vi "MergeFiles.vi"(4 "Error In":errorcluster, 6 "MergeFileConfigIN":T1) -> (0 "sortie d'erreur":errorcluster)   [LabVIEW 2017]
uses:
  DefDeType/WhichPath.ctl
  DefDeType/MergeFileConfig.ctl
panel:
  out "AllWaveForms":waveform(dbl)[](graph)
  out "NortekWaveForms":waveform(dbl)[](graph)
  out "HexapodWaveForms":waveform(dbl)[](graph)
  out "QualisysWaveform":waveform(dbl)[](graph)
  out "ValiseWaveform":waveform(dbl)[](graph)
  out "Etat":string
  # "Merging files"
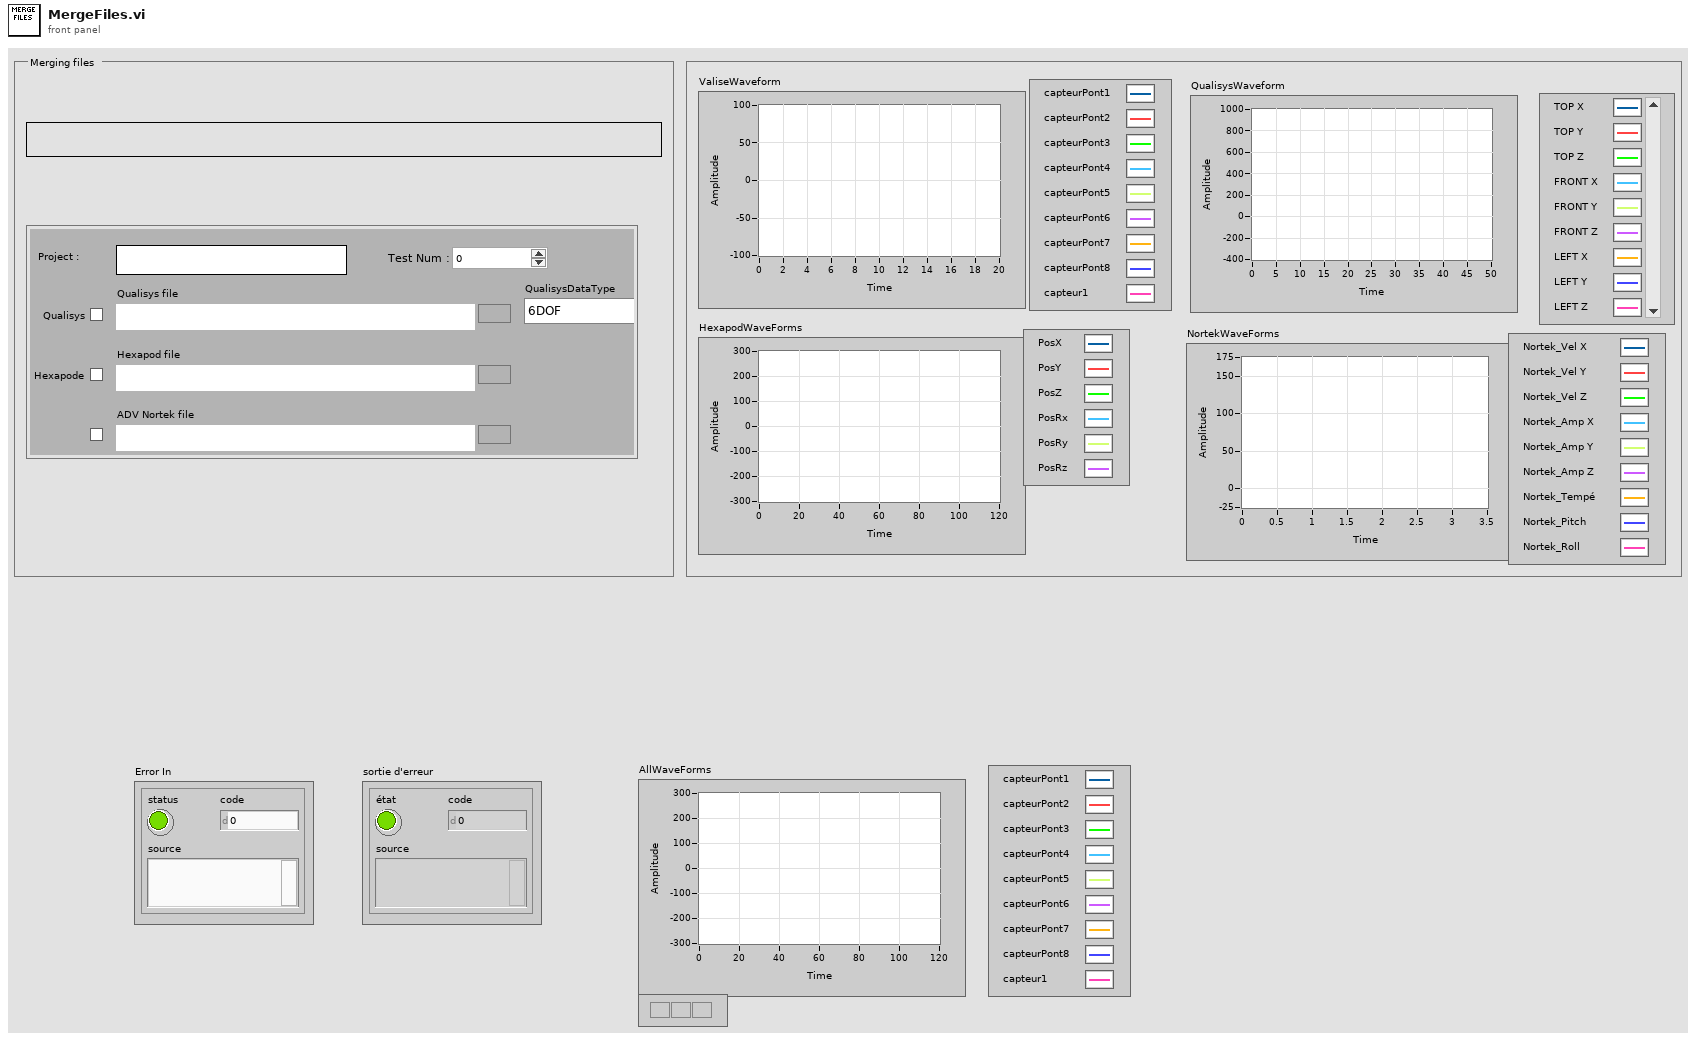
[diagram p1: front panel]
types:
  T1 = typedef "MergeFileConfig.ctl" = cluster{"Test Num : ":u32, "Project :":string, "Qualisys file":path, "Hexapod file":path, "ADV Nortek file":path, "QualisysDataType":enum16{"6DOF", "3DTracking", "6DOF + 3D"}, "Qualisys":bool, "Hexapode":bool, "ADV Nortek":bool}
  T2 = typedef "WhichPath.ctl" = enum16{"DossierProjet", "Config", "Meas", "MeasPCI", "MeasCRIO1", "MeasCRIO2", "MeasQualisys", "MeasHBM", "MeasTDMS", "Fig", "Res"}
  T3 = enum16{"open", "open or create", "create or replace", "create", "open (read-only)"}
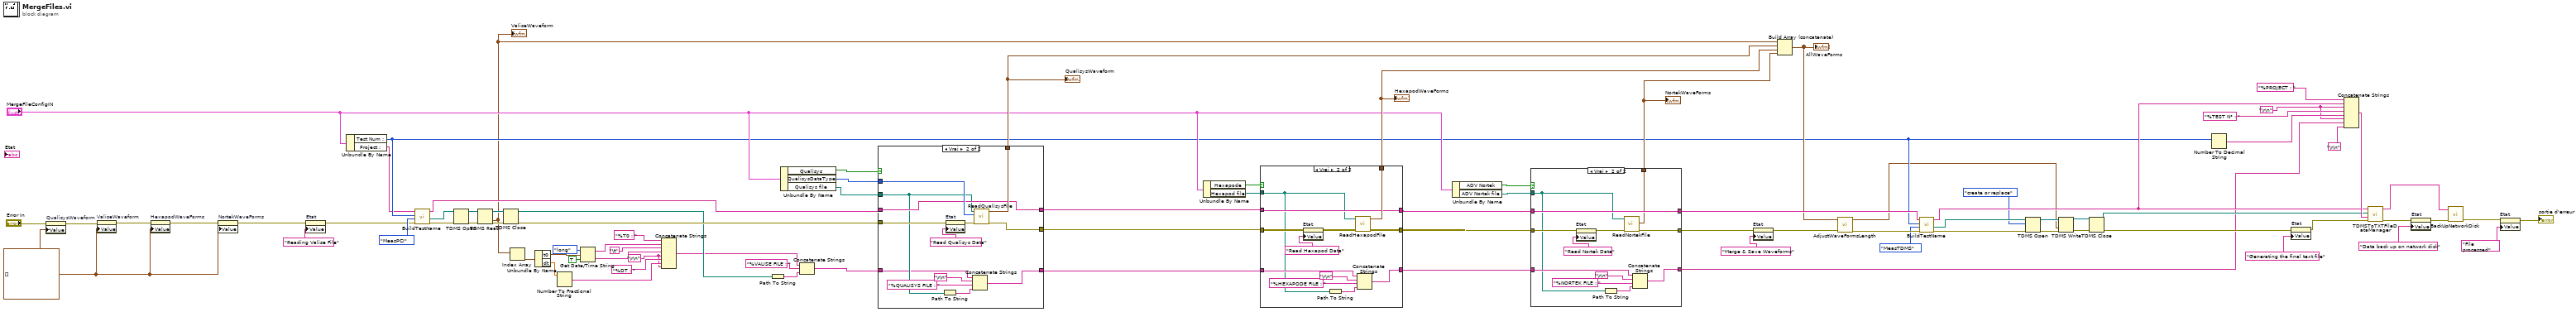
[diagram p0: block diagram]
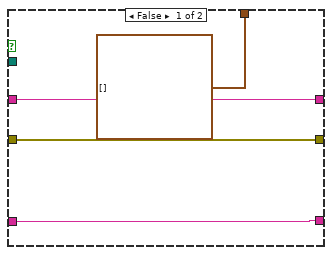
[diagram p2: hidden frame]
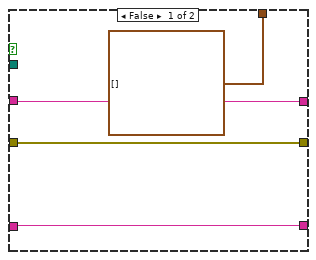
[diagram p3: hidden frame]
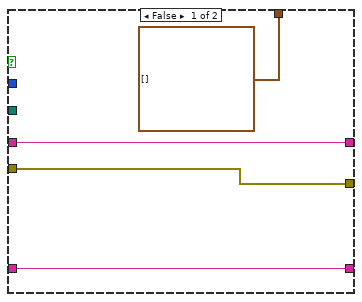
[diagram p4: hidden frame]
diagram:
  w3 = "\r\n"
  w77 = "\r\n"
  w58 = waveform(dbl)[] [] ("QualisysWaveforms")
  n1 = property on="QualisysWaveform" class="GraphWF (strict)"(error in="Error In", "Value"=w58) -> (error out=w82:errorcluster)  [unwired: 1 in, 1 out]
  n2 = property on="ValiseWaveform" class="GraphWF (strict)"(error in=w82, "Value"=w58) -> (error out=w66:errorcluster)  [unwired: 1 in, 1 out]
  n3 = property on="HexapodWaveForms" class="GraphWF (strict)"(error in=w66, "Value"=w58) -> (error out=w59:errorcluster)  [unwired: 1 in, 1 out]
  n4 = property on="NortekWaveForms" class="GraphWF (strict)"(error in=w59, "Value"=w58) -> (error out=w28:errorcluster)  [unwired: 1 in, 1 out]
  n5 = property on="Etat" class="Ch"(error in=w28, "Value"="Reading Valise File" ("Etat")) -> (error out=w29:errorcluster)  [unwired: 1 in, 1 out]
  n6 = Unbundle By Name("MergeFileConfigIN") -> ("Test Num :"=w33:u32, "Project :"=w23:string)
  n7 = call "BuildTestName.vi"("entrée d'erreur"=w29, "WhichPath?"=WhichPath."MeasPCI", "NextTestNum"=w33, "NomProjet"=w23) -> ("sortie d'erreur"=w30:errorcluster, "cheminProchainFichier"=w31:path, "NomProjetOut"=w34:string)  [unwired: 1 in, 1 out]
  n8 = TDMS Open(8:w30, 11:w31) -> (0:w38:errorcluster, 3:w37:refnum<k34>)  [unwired: 5 in]
  n9 = TDMS Read(0:w37, 11:w38) -> (4:w39:refnum<k34>, 10:w15:waveform(dbl)[], 15:w40:errorcluster)  [unwired: 6 in, 3 out]
  "ValiseWaveform" <- w15
  n10 = TDMS Close(8:w40, 11:w39) -> (0:w36:errorcluster, 3:w22:path)
  n11 = Index Array(array=w15) -> (element=w14:waveform(dbl))  [unwired: 1 in]
  n12 = Unbundle By Name(w14) -> ("t0"=w13:timestamp, "dt"=w6:dbl)
  n13 = Number To Fractional String(number=w6) -> (F-format string=w4:string)  [unwired: 3 in]
  n14 = Get Date/Time String(date format (0)=enum16{"short", "long", "abbreviated"}."long", seconds (now)=w13, want seconds? (F)=TRUE) -> (date string=w9:string, time string=w7:string)
  n15 = Concatenate Strings("%T0 : " ("Etat"), w9, "\t", w7, w3, "%DT : " ("Etat"), w4, w3) -> (w2:string)
  n16 = Path To String(path=w22) -> (string=w21:string)
  n17 = Unbundle By Name("MergeFileConfigIN") -> ("Qualisys"=w87:bool, "QualisysDataType"=w86:enum16{"6DOF", "3DTracking", "6DOF + 3D"}, "Qualisys file"=w27:path)
  n18 = Concatenate Strings(w2, "%VALISE FILE : " ("Etat"), w21) -> (w19:string)
  n19 = case shown="Vrai" w87 {
    tunnel: [w91 w105] -> w65
    tunnel: [w92 w99] -> w84
    tunnel: w34 -> [w92 w99]
    tunnel: w36 -> [w91 w100]
    tunnel: w86 -> [_ w104]
    tunnel: [waveform(dbl)[] [] ("QualisysWaveforms") w103] -> w62
    tunnel: w27 -> [_ w96]
    tunnel: w19 -> [w89 w94]
    tunnel: [w89 w93] -> w18
    frame False {
    }
    frame True {
      n20 = Path To String(path=w96) -> (string=w97:string)
      n21 = property on="Etat" class="Ch"(error in=w100, "Value"="Read Qualisys Data" ("Etat")) -> (error out=w101:errorcluster)  [unwired: 1 in, 1 out]
      n22 = Concatenate Strings(w94, "\r\n", "%QUALISYS FILE : " ("Etat"), w97) -> (w93:string)
      n23 = call "ReadQualisysFile.vi"("sortie d'erreur"=w101, "QualisysDataType"=w104, "FichierQualisys"=w96) -> ("error out"=w105:errorcluster, "QualisysWaveforms"=w103:waveform(dbl)[])  [unwired: 3 in]
    }
  }
  "QualisysWaveform" <- w62
  n24 = Unbundle By Name("MergeFileConfigIN") -> ("Hexapode"=w85:bool, "Hexapod file"=w26:path)
  n25 = case shown="Vrai" w85 {
    tunnel: w65 -> [w109 w119]
    tunnel: [w109 w121] -> w63
    tunnel: [w108 w117] -> w64
    tunnel: w84 -> [w108 w117]
    tunnel: [waveform(dbl)[] [] ("QualisysWaveforms") w118] -> w61
    tunnel: w26 -> [_ w111]
    tunnel: w18 -> [w106 w112]
    tunnel: [w106 w110] -> w17
    frame False {
    }
    frame True {
      n26 = property on="Etat" class="Ch"(error in=w119, "Value"="Read Hexapod Data" ("Etat")) -> (error out=w116:errorcluster)  [unwired: 1 in, 1 out]
      n27 = Path To String(path=w111) -> (string=w114:string)
      n28 = call "ReadHexapodFile.vi"("error in (not an error)"=w116, "file path (use dialog)"=w111) -> ("error out"=w121:errorcluster, "WaveformsHexapode"=w118:waveform(dbl)[])  [unwired: 4 in]
      n29 = Concatenate Strings(w112, "\r\n", "%HEXAPODE FILE : " ("Etat"), w114) -> (w110:string)
    }
  }
  "HexapodWaveForms" <- w61
  n30 = Unbundle By Name("MergeFileConfigIN") -> ("ADV Nortek"=w25:bool, "ADV Nortek file"=w24:path)
  n31 = case shown="Vrai" w25 {
    tunnel: w63 -> [w125 w136]
    tunnel: [w125 w135] -> w43
    tunnel: [w124 w133] -> w56
    tunnel: w64 -> [w124 w133]
    tunnel: [waveform(dbl)[] [] ("QualisysWaveforms") w134] -> w60
    tunnel: w24 -> [_ w126]
    tunnel: w17 -> [w122 w128]
    tunnel: [w122 w127] -> w16
    frame False {
    }
    frame True {
      n32 = property on="Etat" class="Ch"(error in=w136, "Value"="Read Nortek Data" ("Etat")) -> (error out=w132:errorcluster)  [unwired: 1 in, 1 out]
      n33 = Path To String(path=w126) -> (string=w130:string)
      n34 = call "ReadNortekFile.vi"("error in"=w132, "FichierNortek"=w126) -> ("error out"=w135:errorcluster, "Nortek WaveForms"=w134:waveform(dbl)[])  [unwired: 4 in]
      n35 = Concatenate Strings(w128, "\r\n", "%NORTEK FILE : " ("Etat"), w130) -> (w127:string)
    }
  }
  "NortekWaveForms" <- w60
  n36 = property on="Etat" class="Ch"(error in=w43, "Value"="Merge & Save Waveforms" ("Etat")) -> (error out=w42:errorcluster)  [unwired: 1 in, 1 out]
  n37 = Build Array (concatenate)(w15, w62, w61, w60) -> (w46:waveform(dbl)[])
  "AllWaveForms" <- w46
  n38 = call "AdjustWaveFormsLength.vi"("error in (no error)"=w42, "AllWaveFormsIN"=w46) -> ("error out"=w57:errorcluster, "AllWaveFormsOUT"=w1:waveform(dbl)[])  [unwired: 4 in]
  n39 = call "BuildTestName.vi"("entrée d'erreur"=w57, "WhichPath?"=WhichPath."MeasTDMS", "NextTestNum"=w33, "NomProjet"=w56) -> ("sortie d'erreur"=w53:errorcluster, "cheminProchainFichier"=w50:path, "NomProjetOut"=w55:string)  [unwired: 1 in, 1 out]
  n40 = TDMS Open(8:w53, 10:T3."create or replace" ("operation (0:open)"), 11:w50) -> (0:w52:errorcluster, 3:w48:refnum<k34>)  [unwired: 4 in]
  n41 = TDMS Write(0:w48, 9:w1, 11:w52) -> (4:w47:refnum<k34>, 15:w51:errorcluster)  [unwired: 3 in, 2 out]
  n42 = TDMS Close(8:w51, 11:w47) -> (0:w45:errorcluster, 3:w41:path)
  n43 = Number To Decimal String(number=w33) -> (decimal integer string=w78:string)  [unwired: 1 in]
  n44 = property on="Etat" class="Ch"(error in=w45, "Value"="Generating the final text file" ("Etat")) -> (error out=w76:errorcluster)  [unwired: 1 in, 1 out]
  n45 = Concatenate Strings("%PROJECT : " ("chaîne"), w55, w77, "%TEST N° : " ("chaîne"), w78, w77, w16, "\r\n") -> (w75:string)
  n46 = call "TDMSToTXTFileDataManager.vi"("entrée d'erreur"=w76, "Info(analog acq,wave,Quali,hexap...)"=w75, "FichierTDMSOrigine"=w41, "NomProj"=w55) -> ("sortie d'erreur"=w71:errorcluster, "NomProjOUT"=w70:string)  [unwired: 1 in, 1 out]
  n47 = property on="Etat" class="Ch"(error in=w71, "Value"="Data back up on network disk" ("Etat")) -> (error out=w72:errorcluster)  [unwired: 1 in, 1 out]
  n48 = call "BackUpNetworkDisk.vi"("Entrée d'erreur"=w72, "NomProjet"=w70) -> ("error out"=w69:errorcluster)  [unwired: 2 in, 1 out]
  n49 = property on="Etat" class="Ch"(error in=w69, "Value"="File processed" ("Etat")) -> (error out=→"sortie d'erreur":errorcluster)  [unwired: 1 in, 1 out]
